vi "RichToFlatni_measurementlink_sessionmanagement_v1_ChannelMapping.vi"(5 "OutputClusterType":T1, 11 "InputCluster":T2) -> (3 "OutputCluster":T1)   [LabVIEW 2021, in "Measurement Plugin Session Management Client.lvlib"]
uses:
  Measurement Plugin Session Management Client.lvlib
  ni_measurementlink_sessionmanagement_v1_ChannelMapping.ctl
  ni_measurementlink_sessionmanagement_v1_ChannelMapping_Flat.ctl
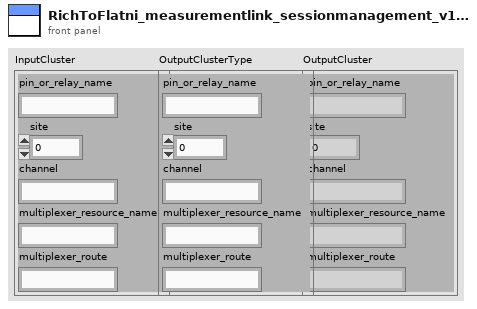
[diagram p1: front panel]
types:
  T1 = typedef "Measurement Plugin Session Management Client.lvlib/ni_measurementlink_sessionmanagement_v1_ChannelMapping_Flat.ctl" = cluster{"pin_or_relay_name":string, "site":i32, "channel":string, "multiplexer_resource_name":string, "multiplexer_route":string}
  T2 = typedef "Measurement Plugin Session Management Client.lvlib/ni_measurementlink_sessionmanagement_v1_ChannelMapping.ctl" = cluster{"pin_or_relay_name":string, "site":i32, "channel":string, "multiplexer_resource_name":string, "multiplexer_route":string}
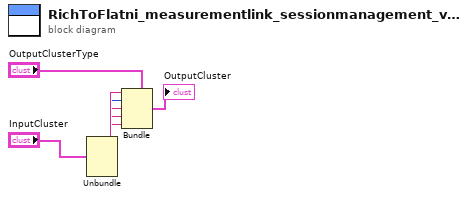
[diagram p0: block diagram]
diagram:
  n1 = Unbundle "Unbundle"("InputCluster") -> ("pin_or_relay_name"=w5:string, "site"=w4:i32, "channel"=w3:string, "multiplexer_resource_name"=w2:string, "multiplexer_route"=w1:string)
  n2 = Bundle "Bundle"(cluster="OutputClusterType", "pin_or_relay_name"=w5, "site"=w4, "channel"=w3, "multiplexer_resource_name"=w2, "multiplexer_route"=w1) -> (→"OutputCluster":T1)
